vi "Reset SMU.vi"(5 "SMU B (No)":bool, 7 "SMU A (No)":bool, 8 "error in (no error)":errorcluster, 10 "Node In":string, 11 "VISA resource name":refnum<visa-resource-name>) -> (0 "error out":errorcluster, 2 "Node Out":string, 3 "VISA resource name out":refnum<visa-resource-name>, 4 "Command String":string)   [LabVIEW 2018, in "Keithley 2600 Series.lvlib"]
doc: "Used to reset SMU A and/or B to their default setups without resetting the entire box.\n\n<b>Functions and Attributes Used</b>\nsmuX.reset()\nX = SMU channel (a or b)"
uses:
  Keithley 2600 Series.lvlib
  Private/GlobalVariables.vi
panel:
  # "(c) 2008 Keithley Instruments, Inc.  ALL RIGHTS RESERVED."
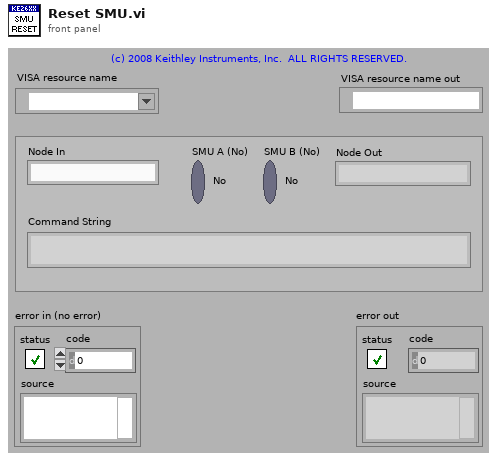
[diagram p1: front panel]
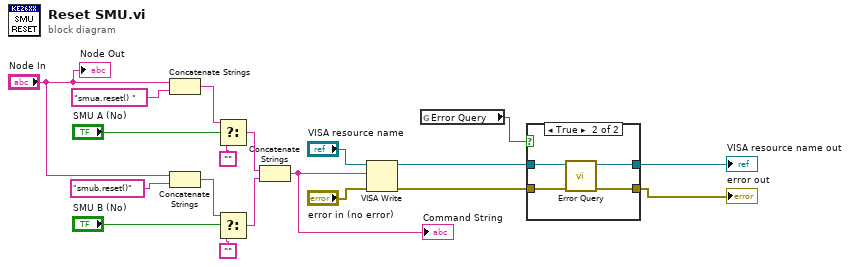
[diagram p0: block diagram]
diagram:
  n1 = Concatenate Strings("Node In", "smua.reset() ") -> (w13:string)
  n2 = Concatenate Strings("Node In", "smub.reset()") -> (w12:string)
  n3 = Select(t=w13, s="SMU A (No)", f="") -> (s? t:f=w11:string)
  n4 = Select(t=w12, s="SMU B (No)", f="") -> (s? t:f=w10:string)
  n5 = Concatenate Strings(w11, w10) -> (w7:string)
  "Command String" <- w7
  n6 = VISA Write(VISA resource name="VISA resource name", write buffer=w7, error in (no error)="error in (no error)") -> (VISA resource name out=w5:refnum<visa-resource-name>, error out=w4:errorcluster)  [unwired: 1 out]
  n7 = global read "GlobalVariables.vi" "Error Query"() -> (w1:bool)
  n8 = case shown="True" w1 {
    tunnel: w5 -> [w21 w25]
    tunnel: w4 -> [w20 w24]
    tunnel: [w21 w23] -> w3
    tunnel: [w20 w22] -> w2
    frame False {
    }
    frame True {
      n9 = call "Error Query.vi"("error in (no error)"=w24, "VISA resource name"=w25) -> ("error out"=w22:errorcluster, "VISA resource name out"=w23:refnum<visa-resource-name>)  [unwired: 8 out]
    }
  }
  "VISA resource name out" <- w3
  "error out" <- w2
  "Node Out" <- "Node In"
